vi "setCanNodeID.vi"(8 "error in (no error)":errorcluster caption="错误输入（无错误）", 10 "CAN node ID":dbl, 11 "StepMotor输入":refnum<class "StepMotor.lvclass">) -> (0 "error out":errorcluster caption="错误输出", 3 "StepMotor输出":refnum<class "StepMotor.lvclass">)   [LabVIEW 2016, in "MotionControl_UFO_3DOF.lvlib" / "StepMotor.lvclass"]
uses:
  <userlib>/MotionControl_UFO_3DOF/StepMotor/StepMotor.lvclass
  <userlib>/MotionControl_UFO_3DOF/StepMotor/StepMotor.lvclass/StepMotor.ctl
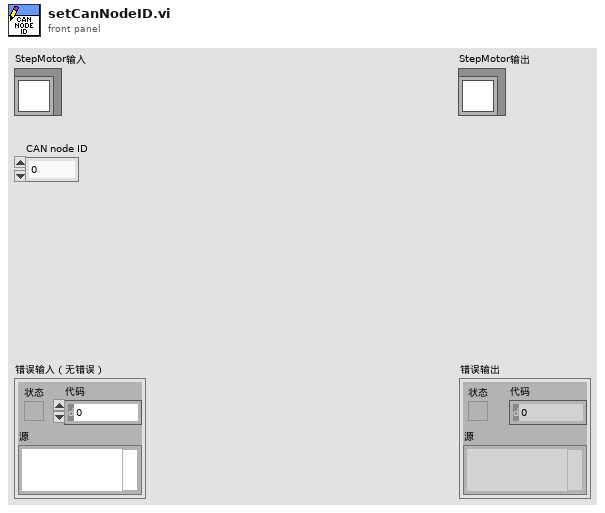
[diagram p1: front panel]
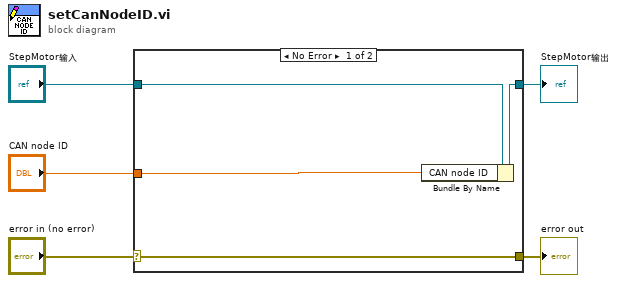
[diagram p0: block diagram]
diagram:
  n1 = case shown="No Error" "error in (no error)" {
    selector: "error in (no error)" -> [w9 w10]
    tunnel: [w9 w10] -> w4
    tunnel: [w7 w11] -> w2
    tunnel: "StepMotor输入" -> [w8 w11]
    tunnel: "CAN node ID" -> [w6 _]
    frame No Error {
      n2 = Bundle By Name(cluster=w8, "CAN node ID"=w6) -> (w7:refnum<class "StepMotor.lvclass">)
    }
    frame Error {
    }
  }
  "error out" <- w4
  "StepMotor输出" <- w2
